vi "roller_map_button_to_state.vi"(10 "Button":bool, 11 "roller user state":T1) -> ()   [LabVIEW 2011]
uses:
  roller_user_state.ctl
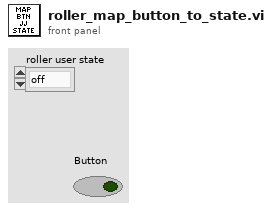
[diagram p1: front panel]
types:
  T1 = typedef "roller_user_state.ctl" = enum16{"off", "collect", "blow"}
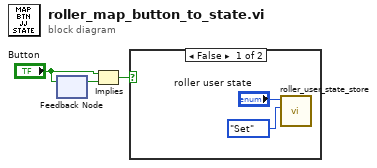
[diagram p0: block diagram]
diagram:
  n1 = feedback-in #1("Button") -> ()
  n2 = feedback #1() -> (w2:bool)  [unwired: 1 in]
  n3 = Implies(1:w2, 2:"Button") -> (0:w1:bool)
  n4 = case shown="False" w1 {
    frame False {
      n5 = call "roller_user_state_store.vi"("data_store_mode"=enum16{"Set", "Get"}."Set", "roller user state"="roller user state") -> ()  [unwired: 9 in, 1 out]
    }
    frame True {
    }
  }
